vi "TPNT_DOAlarm.vi"(4 "mailserver":string="localhost", 5 "tpnt_logfile":path, 6 "tpnt type":string, 7 "next alarm (msecs)":i32, 8 "arguments":string, 9 "device":string, 10 "action":string, 11 "alarm message":string) -> ()   [LabVIEW 2016]
uses:
  DBSHAND/private/vis/DatabaseHand_Element_Get(string).vi
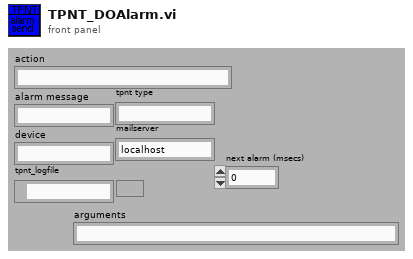
[diagram p1: front panel]
types:
  T1 = typedef "DatabaseHand_RefNum.ctl" = refnum<vi>
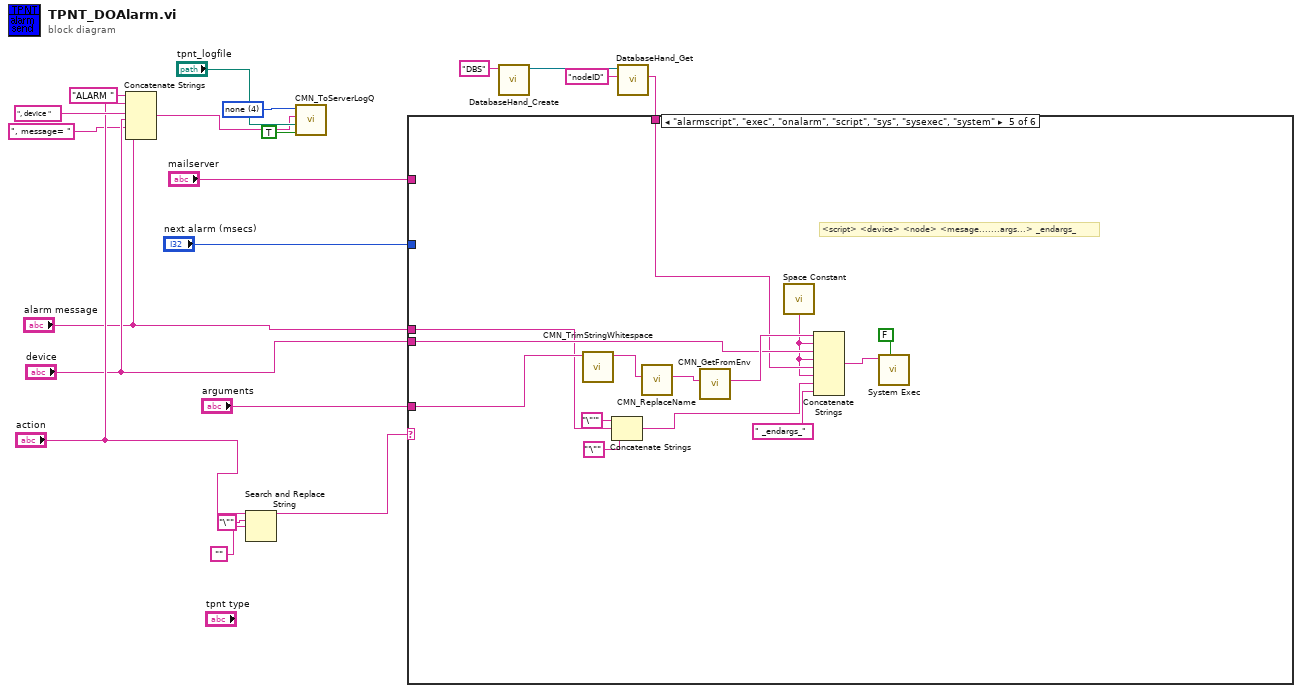
[diagram p0: block diagram]
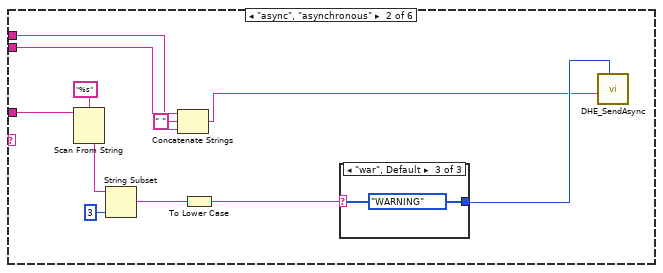
[diagram p3: hidden frame]
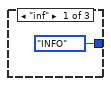
[diagram p4: hidden frame]
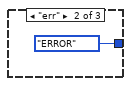
[diagram p5: hidden frame]
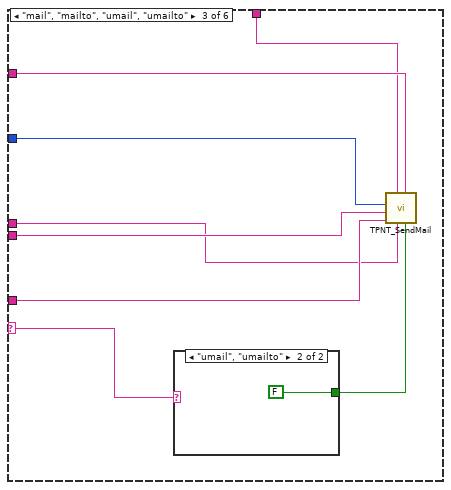
[diagram p6: hidden frame]
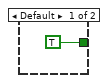
[diagram p7: hidden frame]
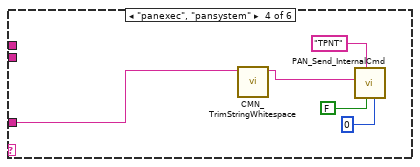
[diagram p8: hidden frame]
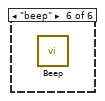
[diagram p9: hidden frame]
diagram:
  w13 = u16 4 items=["command", "imediateReply", "Callback Reply", "Information", "none"] ("type")
  n1 = Concatenate Strings("ALARM " ("string"), "action", ", device " ("string"), "device", ", message= " ("string"), "alarm message") -> (w11:string)
  n2 = Search and Replace String(input string="action", search string="\"", replace string="") -> (result string=w16:string)  [unwired: 1 in, 7 out]
  n3 = call "CMN_ToServerLogQ.vi"("Log"=TRUE, "file"="tpnt_logfile", "string"=w11, "type"=w13) -> ()  [unwired: 2 in, 5 out]
  n4 = call "DatabaseHand_Create.vi"("Name"="DBS") -> ("Database RefNum out"=w3:T1)  [unwired: 1 in, 9 out]
  n5 = call-poly "DatabaseHand_Get.vi"("name"="nodeID", "Database RefNum in"=w3) -> ("value"=w1:string)  [unwired: 3 in, 6 out]
  n6 = case shown="\"alarmscript\", \"exec\", \"onalarm\", \"script\", \"sys\", \"sysexec\", \"system\"" w16 {
    selector: w16 -> [_ _ w37 _ _ _]
    tunnel: "device" -> [_ w25 w41 _ w59 _]
    tunnel: "alarm message" -> [_ w24 w38 _ w53 _]
    tunnel: "arguments" -> [_ w26 w39 w49 w63 _]
    tunnel: "next alarm (msecs)" -> [_ _ w42 _ _ _]
    tunnel: "mailserver" -> [_ _ w40 _ _ _]
    tunnel: w1 -> [_ _ w35 _ w58 _]
    frame Default {
    }
    frame "async", "asynchronous" {
      n7 = Scan From String(format string="%s", input string=w26) -> (output 1=w28:string)  [unwired: 2 in, 4 out]
      n8 = String Subset(string=w28, length (rest)=3 ("length (rest)")) -> (substring=w29:string)  [unwired: 1 out]
      n9 = Concatenate Strings(w25, " " ("string"), w24) -> (w22:string)
      n10 = To Lower Case(string=w29) -> (all lower case string=w21:string)
      n11 = case shown="\"war\", Default" w21 {
        tunnel: [enum16{"ERROR", "WARNING", "INFO", "CHANGED"}."INFO" ("type") enum16{"ERROR", "WARNING", "INFO", "CHANGED"}."ERROR" ("type") enum16{"ERROR", "WARNING", "INFO", "CHANGED"}."WARNING" ("type")] -> w27
        frame "inf" {
        }
        frame "err" {
        }
        frame "war", Default {
        }
      }
      n12 = call "DHE_SendAsync.vi"("type"=w27, "Message"=w22) -> ()  [unwired: 2 in, 8 out]
    }
    frame "mail", "mailto", "umail", "umailto" {
      n13 = case shown="\"umail\", \"umailto\"" w37 {
        tunnel: [TRUE FALSE] -> w36
        frame Default {
        }
        frame "umail", "umailto" {
        }
      }
      n14 = call "TPNT_SendMail.vi"("labmail"=w36, "mailserver"=w40, "alarm message"=w38, "application name"=w35, "arguments"=w39, "device"=w41, "next alarm (msec)"=w42) -> ()  [unwired: 5 out]
    }
    frame "panexec", "pansystem" {
      n15 = call "CMN_TrimStringWhitespace.vi"("string"=w49) -> ("trimmed string"=w48:string)  [unwired: 1 in, 8 out]
      n16 = call "PAN_Send_InternalCmd.vi"("timeout in ms (-1)"=0, "wait response"=FALSE, "taskID"="TPNT", "command"=w48) -> ()  [unwired: 1 in, 7 out]
    }
    frame "alarmscript", "exec", "onalarm", "script", "sys", "sysexec", "system" {
      # "<script> <device> <node> <mesage.......args...> _endargs_"
      n17 = call "CMN_TrimStringWhitespace.vi"("string"=w63) -> ("trimmed string"=w55:string)  [unwired: 1 in, 8 out]
      n18 = Concatenate Strings("\"'" ("string"), w53, "'\"" ("string")) -> (w52:string)
      n19 = call "CMN_ReplaceName.vi"("name in"=w55) -> ("name out"=w54:string)  [unwired: 1 in, 9 out]
      n20 = call "CMN_GetFromEnv.vi"("str in"=w54) -> ("str out"=w61:string)  [unwired: 10 out]
      n21 = call <vilib>:"Space Constant.vi"() -> ("String"=w57:string)
      n22 = Concatenate Strings(w61, w57, w59, w57, w58, w57, w52, " _endargs_" ("string")) -> (w60:string)
      n23 = call <vilib>:"System Exec.vi"("wait until completion? (T)"=FALSE, "command line"=w60) -> ()  [unwired: 4 in, 6 out]
    }
    frame "beep" {
      n24 = call <vilib>:"Beep.vi"() -> ()  [unwired: 3 in, 9 out]
    }
  }
